vi "ASM182T_Read.vi"(1 "Pump Address":refnum<visa-resource-name>) -> (0 "HELIUM LEVEL":dbl format="%#.1e")   [LabVIEW 2019]
panel:
  out "Pressure out":variant
  out "error out":errorcluster
  in  "stop":bool
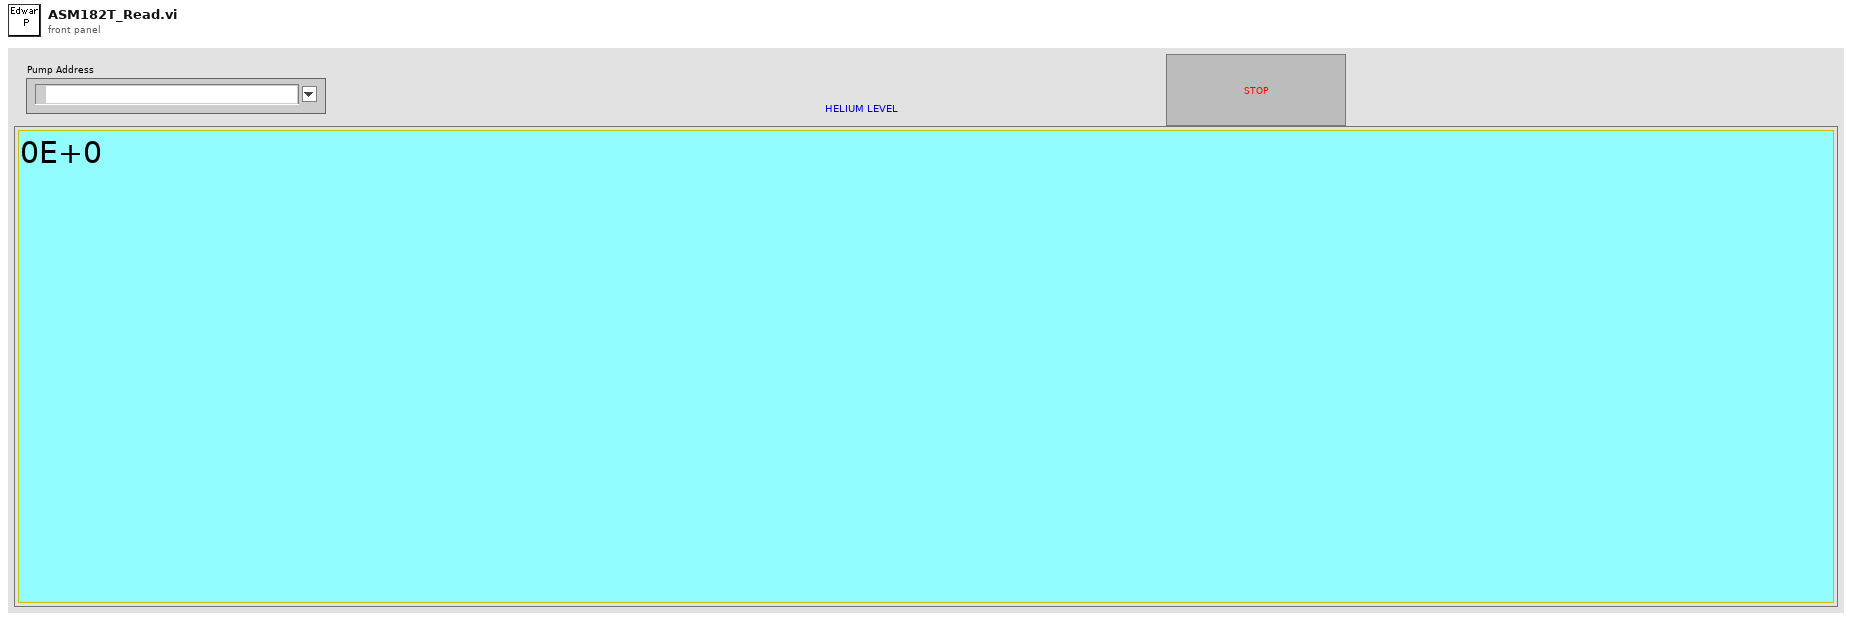
[diagram p1: front panel]
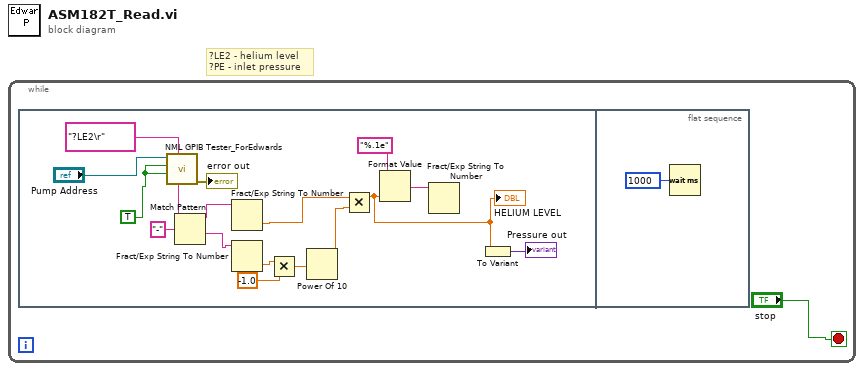
[diagram p0: block diagram]
diagram:
  # "?LE2 - helium level\n?PE - inlet pressure"
  n1 = while {
    stop <- "stop" stop-if-true
    n2 = flat-sequence {
      frame #0 {
        w15 = TRUE ("Write")
        n3 = call "NML GPIB Tester_ForEdwards.vi"(5:"?LE2\r", "Read"=w15, "Write"=w15, "VISA resource name"="Pump Address") -> ("error out"=→"error out":errorcluster, 4:w11:string)  [unwired: 4 in]
        n4 = Match Pattern(string=w11, regular expression="-") -> (before substring=w7:string, after substring=w8:string)  [unwired: 1 in, 2 out]
        n5 = Fract/Exp String To Number(string=w7) -> (number=w4:dbl)  [unwired: 3 in, 1 out]
        n6 = Fract/Exp String To Number(string=w8) -> (number=w6:dbl)  [unwired: 3 in, 1 out]
        n7 = Multiply(x=w6, y=-1.0) -> (x*y=w10:dbl)
        n8 = Power Of 10(x=w10) -> (10^x=w9:dbl)
        n9 = Multiply(x=w4, y=w9) -> (x*y=w2:dbl)
        "HELIUM LEVEL" <- w2
        n10 = Format Value(format string="%.1e", value (0)=w2) -> (output string=w3:string)  [unwired: 1 in]
        n11 = Fract/Exp String To Number(string=w3) -> ()  [unwired: 3 in, 2 out]
        n12 = To Variant(anything=w2) -> (Variant=→"Pressure out":variant)
      }
      frame #1 {
        n13 = Wait (ms)(milliseconds to wait=u32 1000) -> ()  [unwired: 1 out]
      }
    }
  }
